vi "createNewArrayObject.vi"(8 "error in (no error)":errorcluster, 10 "arrayRef":refnum<vi>, 11 "UnsignedShort in":refnum<class "UnsignedShort.lvclass">) -> (0 "error out":errorcluster, 3 "UnsignedShort out":refnum<class "UnsignedShort.lvclass">)   [LabVIEW 2013, in "UnsignedShort.lvclass"]
uses:
  UnsignedShort.lvclass
  <vilib>/numeric/LVNumericRepresentation.ctl
  Numeric/Numeric.lvclass/Numeric.ctl
  Unsigned/Unsigned.lvclass
  Numeric/Numeric.lvclass
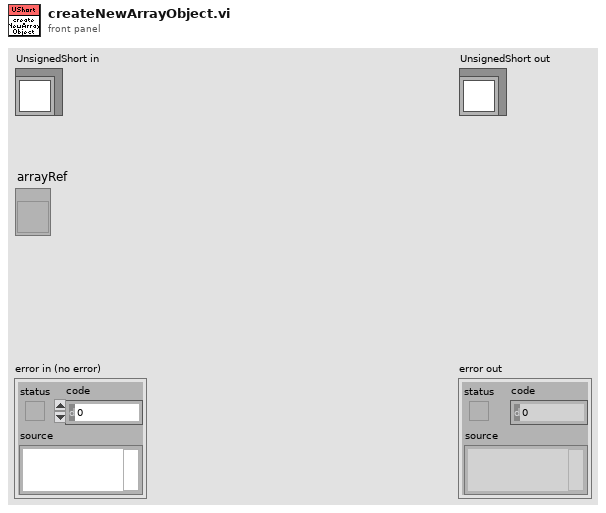
[diagram p1: front panel]
types:
  T1 = typedef "LVNumericRepresentation.ctl" = enum32{"Extended Precision", "Double Precision", "Single Precision", "Long", "Word", "Byte", "Unsigned Long", "Unsigned Word", "Unsigned Byte", "Complex Extended", "Complex Double", "Complex Single", "Quad", "Unsigned Quad", "Fixed-Point"}
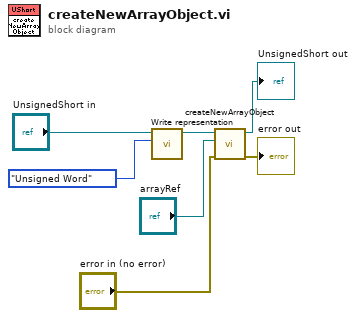
[diagram p0: block diagram]
diagram:
  n1 = call "Write representation.vi"("Numeric Representation"=LVNumericRepresentation."Unsigned Word", "Numeric in"="UnsignedShort in") -> ("Numeric out"=w2:refnum<class "UnsignedShort.lvclass">)  [unwired: 9 in]
  n2 = call-parent "createNewArrayObject.vi"("error in (no error)"="error in (no error)", "arrayRef"="arrayRef", "Numeric in"=w2) -> ("error out"=→"error out":errorcluster, "Numeric out"=→"UnsignedShort out":refnum<class "UnsignedShort.lvclass">)  [unwired: 7 in]
